vi "ColorAPI_Init.vi"(8 "错误输入（无错误）":errorcluster, 11 "端口号":i32) -> (0 "错误输出":errorcluster, 2 "返回值":bool, 3 "端口号输出":i32)   [LabVIEW 2011, in "ColorSensorlib.lvlib"]
uses:
  ColorSensorlib.lvlib
  ColorDis.dll
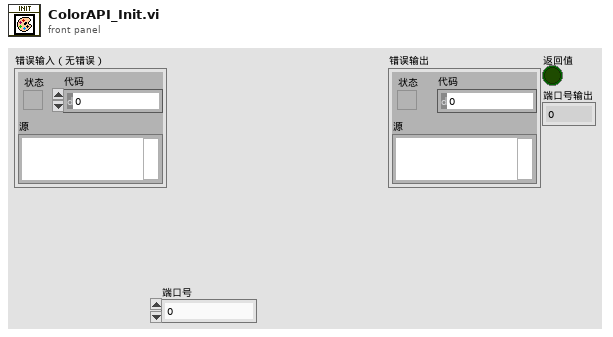
[diagram p1: front panel]
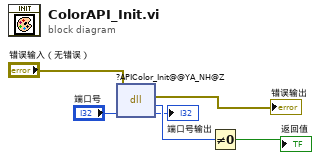
[diagram p0: block diagram]
diagram:
  n1 = dll-call lib="PTH1Cabs D\tDocumentsDesktop颜色传感器LabViewColorDis.dll" fn="?APIColor_Init@@YA_NH@Z"(error in="错误输入（无错误）", "Com"="端口号") -> (error out=→"错误输出":errorcluster, "Rtv"=w3:i32, "Com"=→"端口号输出":i32)  [unwired: 2 in, 1 out]
  n2 = Not Equal To 0?(x=w3) -> (x != 0?=→"返回值":bool)
